vi "Run.vi"(8 "error in (no error)":errorcluster, 11 "socket REQ in":refnum<class "socket REQ.lvclass">) -> (0 "error out":errorcluster, 3 "socket REQ out":refnum<class "socket REQ.lvclass">)   [LabVIEW 2018, in "socket REQ.lvclass"]
uses:
  socket REQ.lvclass
  C:/Users/devstaff/sparc4/s4gui/Versao ZeroMQ REQ-REP/SPARC4_GUI -v1.0.8 - com pacote communication manager/communication-manager/Socket/Socket.lvclass
  Socket/Socket.lvclass
  State Machine/CM_State Machine.lvclass
  RxTx/CM_RxTx.lvclass
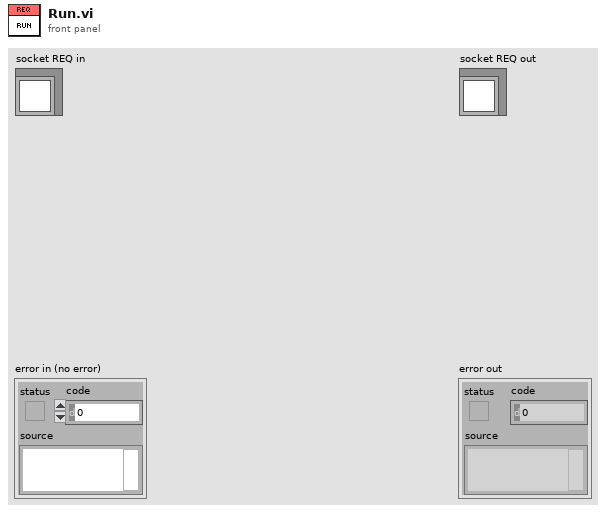
[diagram p1: front panel]
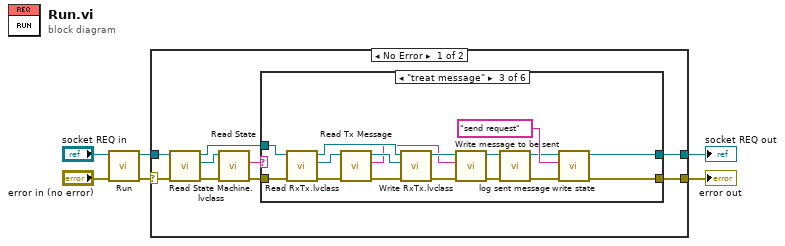
[diagram p0: block diagram]
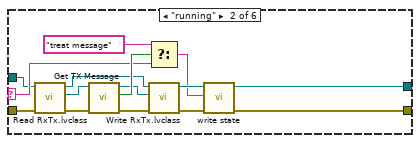
[diagram p3: hidden frame]
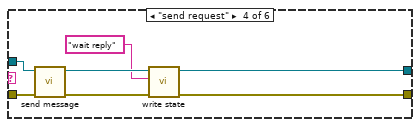
[diagram p4: hidden frame]
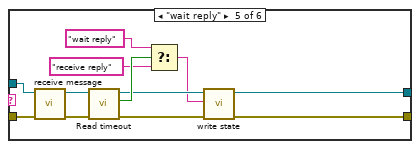
[diagram p5: hidden frame]
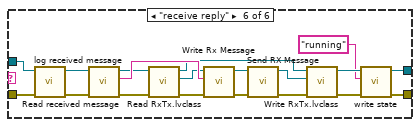
[diagram p6: hidden frame]
diagram:
  n1 = call-parent "Run.vi"("error in (no error)"="error in (no error)", "Socket in"="socket REQ in") -> ("error out"=w3:errorcluster, "Socket out"=w4:refnum<class "socket REQ.lvclass">)  [unwired: 8 in]
  n2 = case shown="No Error" w3 {
    selector: w3 -> [w11 w88]
    tunnel: w4 -> [w9 w89]
    tunnel: [w7 w89] -> w2
    tunnel: [w10 w88] -> w1
    frame No Error {
      n3 = call-dynamic "Read State Machine.lvclass.vi"("error in (no error)"=w11, "Socket in"=w9) -> ("error out"=w13:errorcluster, "State Machine.lvclass"=w15:refnum<class "CM_State Machine.lvclass">, "Socket out"=w8:refnum<class "socket REQ.lvclass">)  [unwired: 7 in]
      n4 = call-dynamic "Read State.vi"("error in (no error)"=w13, "State Machine in"=w15) -> ("error out"=w12:errorcluster, "State"=w14:string)  [unwired: 7 in, 1 out]
      n5 = case shown="\"treat message\"" w14 {
        selector: w14 -> [_ w31 _ _ _ _]
        tunnel: w8 -> [w17 w24 w49 w56 w67 w69]
        tunnel: [w17 w21 w34 w54 w58 w76] -> w7
        tunnel: [w16 w20 w33 w53 w59 w75] -> w10
        tunnel: w12 -> [w16 w29 w48 w50 w68 w70]
        frame Default {
        }
        frame "running" {
          n6 = call-dynamic "Read RxTx.lvclass.vi"("error in (no error)"=w29, "Socket in"=w24) -> ("error out"=w26:errorcluster, "RxTx.lvclass"=w28:refnum<class "CM_RxTx.lvclass">, "Socket out"=w23:refnum<class "socket REQ.lvclass">)  [unwired: 7 in]
          n7 = call "Get TX Message.vi"("error in (no error)"=w26, "RxTx in"=w28) -> ("error out"=w25:errorcluster, "New msg"=w32:bool, "RxTx out"=w27:refnum<class "CM_RxTx.lvclass">)  [unwired: 7 in]
          n8 = Select(t="treat message", s=w32, f=w31) -> (s? t:f=w18:string)
          n9 = call-dynamic "Write RxTx.lvclass.vi"("error in (no error)"=w25, "RxTx.lvclass"=w27, "Socket in"=w23) -> ("error out"=w19:errorcluster, "Socket out"=w22:refnum<class "socket REQ.lvclass">)  [unwired: 7 in]
          n10 = call "write state.vi"("error in (no error)"=w19, "State"=w18, "Socket in"=w22) -> ("error out"=w20:errorcluster, "Socket out"=w21:refnum<class "socket REQ.lvclass">)  [unwired: 7 in]
        }
        frame "treat message" {
          n11 = call-dynamic "Read RxTx.lvclass.vi"("error in (no error)"=w48, "Socket in"=w49) -> ("error out"=w41:errorcluster, "RxTx.lvclass"=w47:refnum<class "CM_RxTx.lvclass">, "Socket out"=w46:refnum<class "socket REQ.lvclass">)  [unwired: 7 in]
          n12 = call "Read Tx Message.vi"("error in (no error)"=w41, "RxTx in"=w47) -> ("error out"=w43:errorcluster, "Tx Message"=w35:string, "RxTx out"=w42:refnum<class "CM_RxTx.lvclass">)  [unwired: 7 in]
          n13 = call-dynamic "Write RxTx.lvclass.vi"("error in (no error)"=w43, "RxTx.lvclass"=w42, "Socket in"=w46) -> ("error out"=w44:errorcluster, "Socket out"=w45:refnum<class "socket REQ.lvclass">)  [unwired: 7 in]
          n14 = call-dynamic "Write message to be sent.vi"("error in (no error)"=w44, "message to be sent"=w35, "Socket in"=w45) -> ("error out"=w36:errorcluster, "Socket out"=w39:refnum<class "socket REQ.lvclass">)  [unwired: 7 in]
          n15 = call "log sent message.vi"("error in (no error)"=w36, "Socket in"=w39) -> ("error out"=w37:errorcluster, "Socket out"=w38:refnum<class "socket REQ.lvclass">)  [unwired: 8 in]
          n16 = call "write state.vi"("error in (no error)"=w37, "State"="send request" ("new state"), "Socket in"=w38) -> ("error out"=w33:errorcluster, "Socket out"=w34:refnum<class "socket REQ.lvclass">)  [unwired: 7 in]
        }
        frame "send request" {
          n17 = call "send message.vi"("error in (no error)"=w50, "Socket in"=w56) -> ("error out"=w52:errorcluster, "Socket out"=w55:refnum<class "socket REQ.lvclass">)  [unwired: 8 in]
          n18 = call "write state.vi"("error in (no error)"=w52, "State"="wait reply" ("new state"), "Socket in"=w55) -> ("error out"=w53:errorcluster, "Socket out"=w54:refnum<class "socket REQ.lvclass">)  [unwired: 7 in]
        }
        frame "wait reply" {
          n19 = call-dynamic "receive message.vi"("error in (no error)"=w68, "Socket in"=w67) -> ("error out"=w65:errorcluster, "Socket out"=w66:refnum<class "socket REQ.lvclass">)  [unwired: 8 in]
          n20 = call-dynamic "Read timeout.vi"("error in (no error)"=w65, "Socket in"=w66) -> ("error out"=w60:errorcluster, "timeout"=w64:bool, "Socket out"=w61:refnum<class "socket REQ.lvclass">)  [unwired: 7 in]
          n21 = Select(t="wait reply" ("new state"), s=w64, f="receive reply" ("new state")) -> (s? t:f=w57:string)
          n22 = call "write state.vi"("error in (no error)"=w60, "State"=w57, "Socket in"=w61) -> ("error out"=w59:errorcluster, "Socket out"=w58:refnum<class "socket REQ.lvclass">)  [unwired: 7 in]
        }
        frame "receive reply" {
          n23 = call "log received message.vi"("error in (no error)"=w70, "Socket in"=w69) -> ("error out"=w71:errorcluster, "Socket out"=w72:refnum<class "socket REQ.lvclass">)  [unwired: 8 in]
          n24 = call-dynamic "Read received message.vi"("error in (no error)"=w71, "Socket in"=w72) -> ("error out"=w79:errorcluster, "received message"=w87:string, "Socket out"=w80:refnum<class "socket REQ.lvclass">)  [unwired: 7 in]
          n25 = call-dynamic "Read RxTx.lvclass.vi"("error in (no error)"=w79, "Socket in"=w80) -> ("error out"=w78:errorcluster, "RxTx.lvclass"=w84:refnum<class "CM_RxTx.lvclass">, "Socket out"=w83:refnum<class "socket REQ.lvclass">)  [unwired: 7 in]
          n26 = call "Write Rx Message.vi"("error in (no error)"=w78, "Rx Message"=w87, "RxTx in"=w84) -> ("error out"=w85:errorcluster, "RxTx out"=w86:refnum<class "CM_RxTx.lvclass">)  [unwired: 7 in]
          n27 = call "Send RX Message.vi"("error in (no error)"=w85, "RxTx in"=w86) -> ("error out"=w81:errorcluster, "RxTx out"=w82:refnum<class "CM_RxTx.lvclass">)  [unwired: 8 in]
          n28 = call-dynamic "Write RxTx.lvclass.vi"("error in (no error)"=w81, "RxTx.lvclass"=w82, "Socket in"=w83) -> ("error out"=w74:errorcluster, "Socket out"=w77:refnum<class "socket REQ.lvclass">)  [unwired: 7 in]
          n29 = call "write state.vi"("error in (no error)"=w74, "State"="running" ("new state"), "Socket in"=w77) -> ("error out"=w75:errorcluster, "Socket out"=w76:refnum<class "socket REQ.lvclass">)  [unwired: 7 in]
        }
      }
    }
    frame Error {
    }
  }
  "error out" <- w1
  "socket REQ out" <- w2
